vi "Globals.vi"() -> ()   [LabVIEW 2021]
uses:
  Actors/Alarm Handler/API/Alarm Handler Actor API.lvclass
  Actors/Main Controller/API/Main Controller Actor API.lvclass
  Re-use Libraries/Minimal Actor Framework/Actors/Base Actor/API/Actor API.lvclass
  Actors/Task Scheduler/API/Task Scheduler Actor API.lvclass
  Resource Manager/Resource Manager.lvclass
  Element/Element.lvclass
panel:
  in  "Elements":refnum<class "Element.lvclass">[](array[class])
  in  "Player 2 Inputs":T1
  in  "Resource Manager":refnum<data-value>
  out "About Window":refnum<class "Actor API.lvclass">
  in  "Task Scheduler":refnum<class "Task Scheduler Actor API.lvclass">
  in  "Launcher":refnum<class "Actor API.lvclass">
  in  "Main Controller":refnum<class "Main Controller Actor API.lvclass">
  in  "Alarm Handler":refnum<class "Alarm Handler Actor API.lvclass">
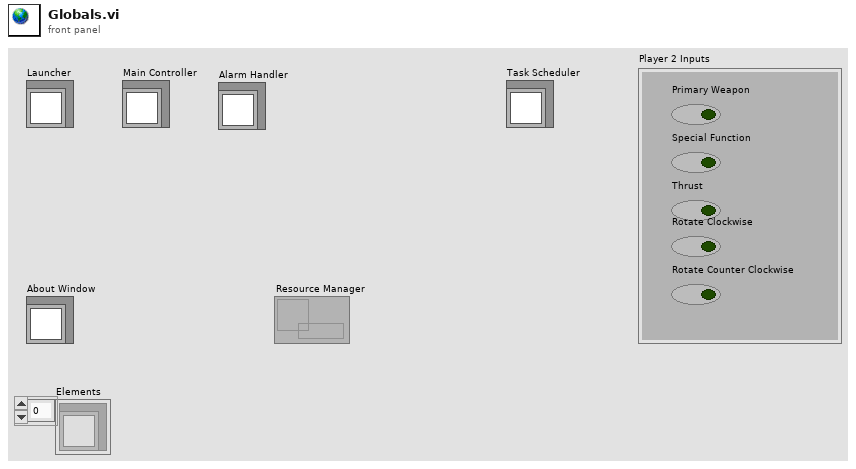
[diagram p1: front panel]
types:
  T1 = cluster{"Primary Weapon":bool, "Special Function":bool, "Thrust":bool, "Rotate Clockwise":bool, "Rotate Counter Clockwise":bool}
diagram:
